vi "MB_Master.vi"() -> ()   [LabVIEW 2015]
doc: "Modbus主机模式"
uses:
  lib/pcomm/PCOMM.lvlib
panel:
  in  "轮询？":bool
  in  "轮询间隔时间":u32=1000 caption="ms" min=30 max=65535 format="%5.0f"
  in  "超时时间":u32=200 caption="ms" min=30 max=65535 format="%5.0f"
  in  "字节数":u16 caption="寄存器值" format="%04x"
  out "LRC8":u8 format="%02x"
  out "CRC16 Hi":u8 format="%02x"
  out "CRC16 Lo":u8 format="%02x"
  in  "数据量":u16 min=1 max=125 format="%04x"
  in  "起始地址":u16 format="%04x"
  in  "功能码":u8(ring)=1 items=["01"=1, "02"=2, "03"=3, "04"=4, "05"=5, "06"=6, "0F"=15, "10"=16]
  in  "从设备编号":u8 format="%02x"
  in  "数据域":u8[](array[numeric]) format="%02x"
  in  "手动发送":bool
  out "接收":string caption="Rx:"
  in  "发送":string caption="Tx:"
  in  "刷新按钮":bool
  in  "字符串":string="串口设置"
  in  "串口号":i32(ring)=1 items=["COM1 通信端口 (COM1)"=1, "COM2 ELTIMA Virtual Serial Port (COM2->COM3)"=2, "COM3 ELTIMA Virtual Serial Port (COM3->COM2)"=3, "COM8 USB-SERIAL CH340 (COM8)"=8]
  in  "奇偶校验":i32(ring)=8 caption="校   验" items=["None"=0, "Odd"=8, "Even"=24, "Mark"=40, "Space"=56]
  in  "数据比特":i32(ring)=3 caption="数据位" items=["5", "6", "7", "8"]
  in  "波特率":i32(ring)=16 items=["1800"=8, "2400"=9, "4800"=10, "7200"=11, "9600"=12, "19200"=13, "38400"=14, "57600"=15, "115200"=16, "230400"=17, "460800"=18, "921600"=19]
  in  "停止位":i32(ring) items=["1"=0, "2"=4]
  in  "打开/关闭串口":bool
  in  "Rx":u32
  in  "Tx":u32
  in  "通信模式":enum16{"RTU", "ASCII"}(ring)
  in  "主从选择":enum32{"Master"}(ring)
  in  "接收帧分析":string
  # "RTU模式不会去检测字符间超时事件"
  # "轮询间隔"
  # "超时时间"
  # "主从模式"
  # "通信模式"
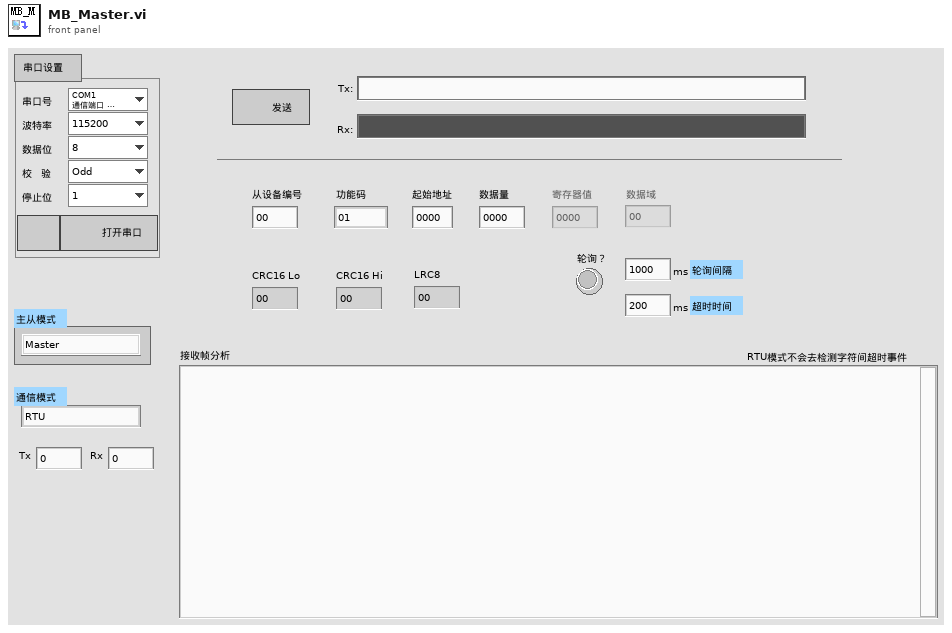
[diagram p1: front panel]
types:
  T1 = enum8{"Enabled", "Disabled", "Disabled and Grayed Out"}
  T2 = typedef "LVRectTypeDef.ctl" = cluster{"Left":i16, "Top":i16, "Right":i16, "Bottom":i16}
  T3 = typedef "LVPointTypeDef.ctl" = cluster{"Horizontal":i16, "Vertical":i16}
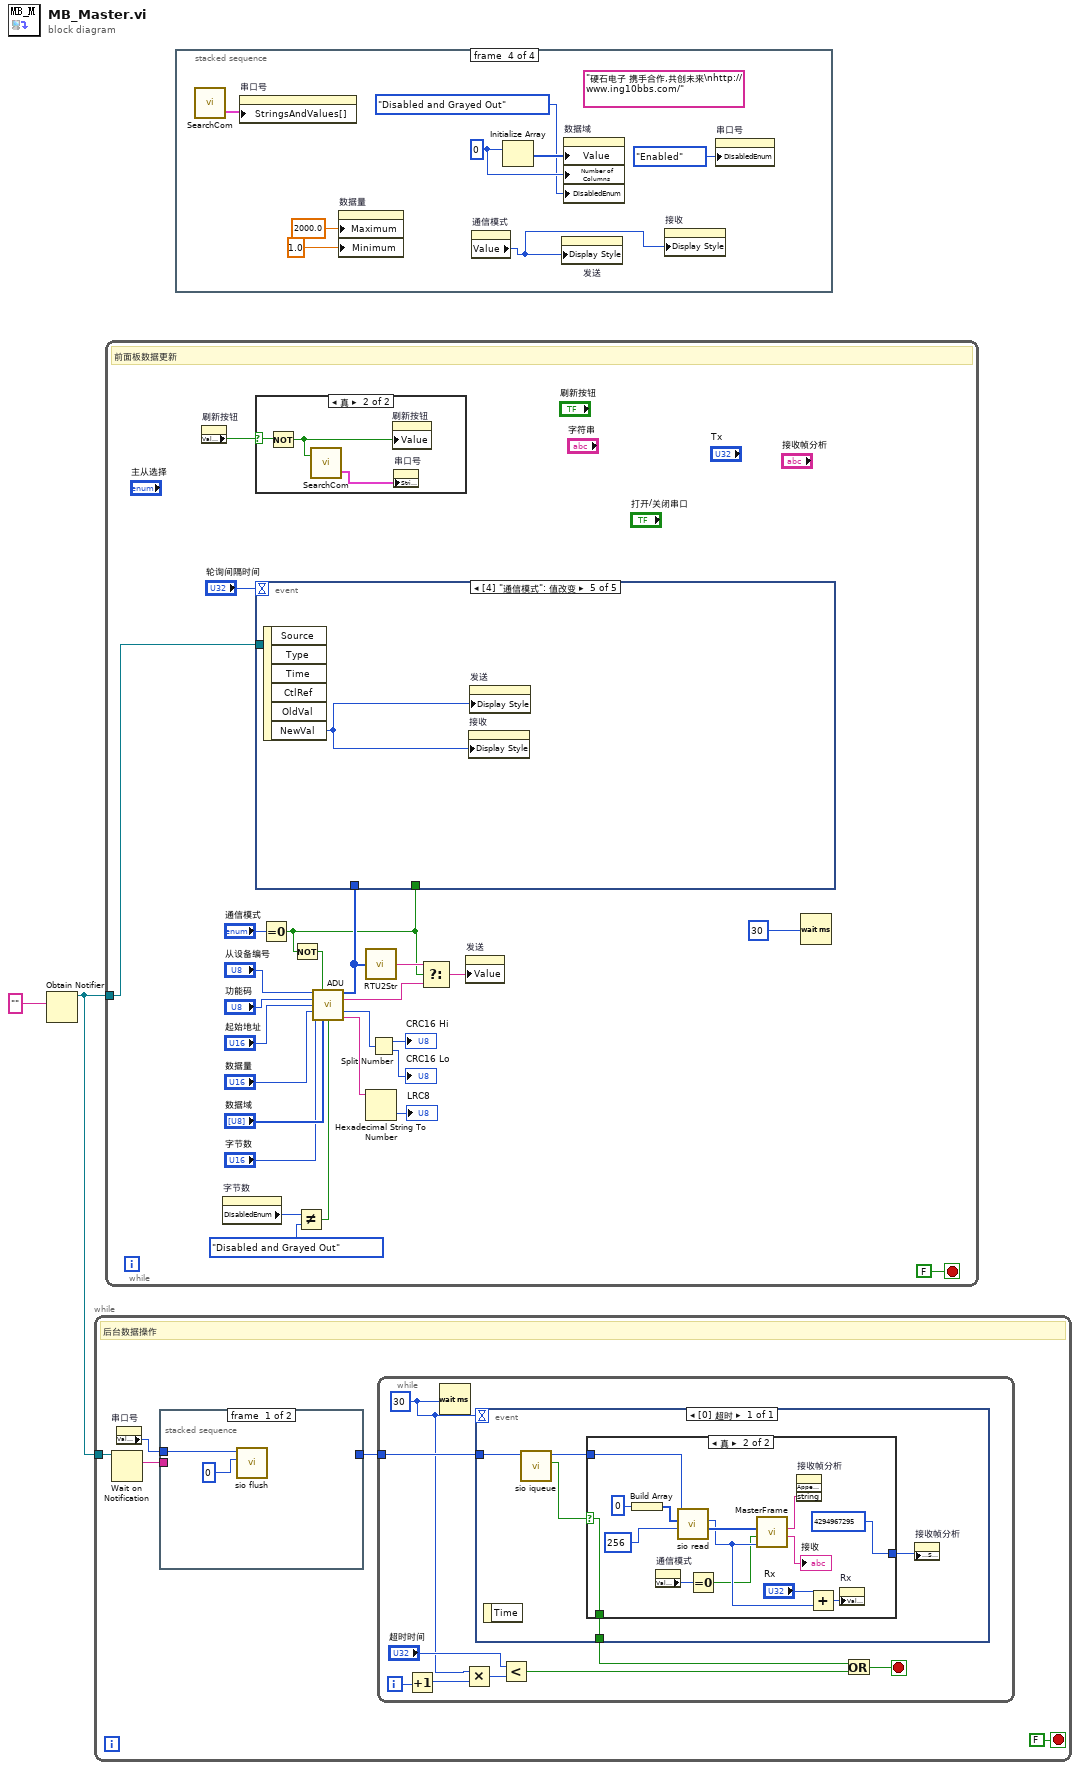
[diagram p0: block diagram]
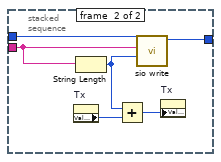
[diagram p2: hidden frame]
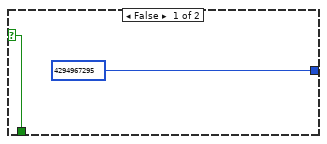
[diagram p3: hidden frame]
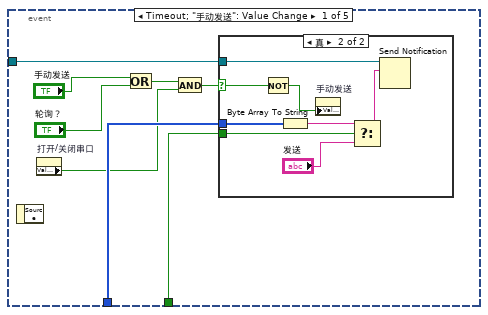
[diagram p4: hidden frame]
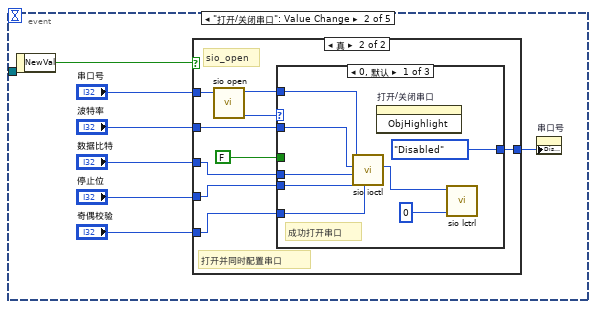
[diagram p6: hidden frame]
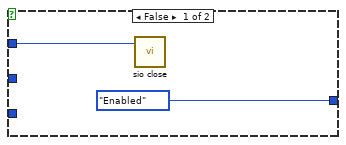
[diagram p7: hidden frame]
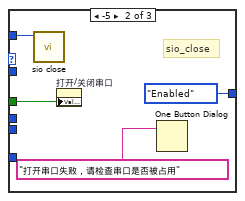
[diagram p8: hidden frame]
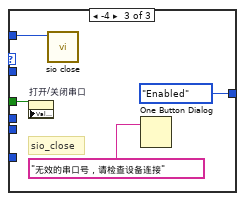
[diagram p9: hidden frame]
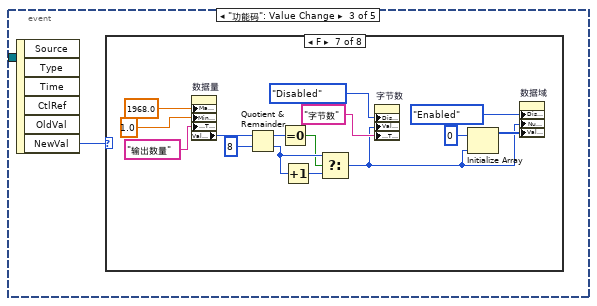
[diagram p10: hidden frame]
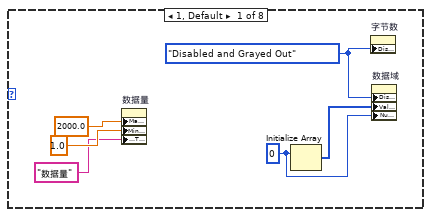
[diagram p11: hidden frame]
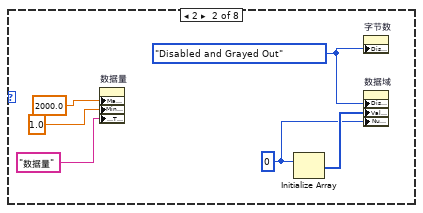
[diagram p12: hidden frame]
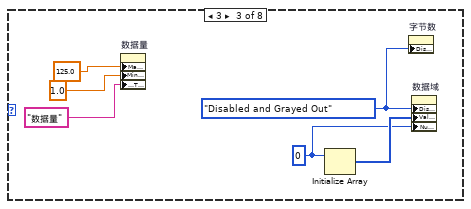
[diagram p13: hidden frame]
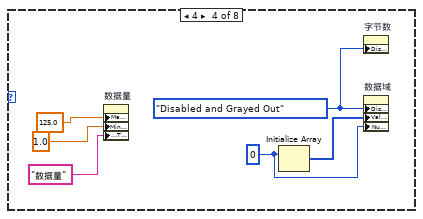
[diagram p14: hidden frame]
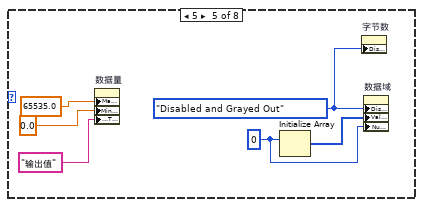
[diagram p15: hidden frame]
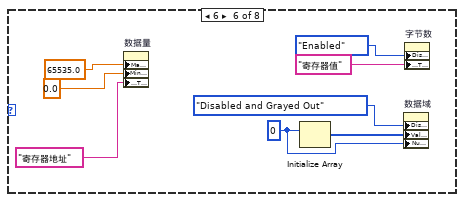
[diagram p16: hidden frame]
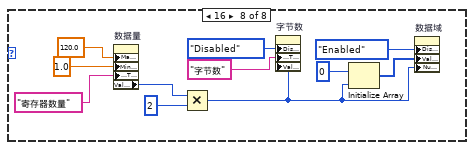
[diagram p17: hidden frame]
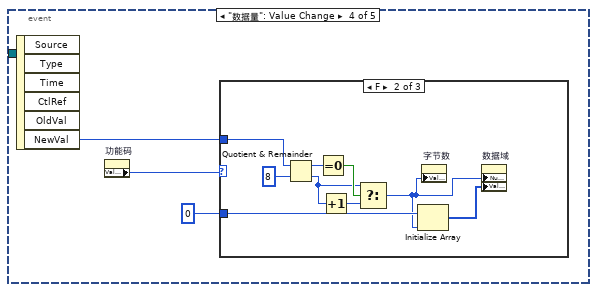
[diagram p18: hidden frame]
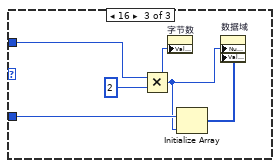
[diagram p20: hidden frame]
diagram:
  n1 = Obtain Notifier(notification data type="") -> (notifier out=w2:refnum<notifier>)  [unwired: 3 in, 2 out]
  n2 = while {
    tunnel: w2 -> [w7]
    stop <- FALSE stop-if-true
    # "后台数据操作"
    n3 = Wait on Notification(notifier=w7) -> (notification=w5:string)  [unwired: 3 in, 3 out]
    n4 = property on="串口号" class="Ring (严格)"() -> ("Value"=w3:i32)  [unwired: 2 in, 2 out]
    n5 = stacked-sequence {
      tunnel: w5 -> [_ w14]
      tunnel: [_ w15] -> w4
      tunnel: w3 -> [w8 w13]
      frame #0 {
        n6 = call "sio flush.vi"("func"=0, "port"=w8) -> ()  [unwired: 8 in, 2 out]
      }
      frame #1 {
        n7 = property on="Tx" class="DigNum (严格)"() -> ("Value"=w11:u32)  [unwired: 2 in, 2 out]
        n8 = String Length(string=w14) -> (length=w12:i32)
        n9 = Add(x=w12, y=w11) -> (x+y=w10:u32)
        n10 = call "sio write.vi"("len"=w12, "buf"=w14, "port"=w13) -> ("port out"=w15:i32)  [unwired: 6 in, 2 out]
        n11 = property on="Tx" class="DigNum (严格)"("Value"=w10) -> ()  [unwired: 2 in, 2 out]
      }
    }
    n12 = while {
      tunnel: w4 -> [w23]
      i -> [w22]
      stop <- w24 stop-if-true
      w16 = 30
      n13 = Increment(x=w22) -> (x+1=w21:i32)
      n14 = Wait (ms)(milliseconds to wait=w16) -> ()  [unwired: 1 out]
      n15 = Multiply(x=w16, y=w21) -> (x*y=w19:i32)
      n16 = event shown="[0] 超时" {
        selector: _ -> [_]
        dyn-events: _ -> [_]
        timeout: w16 -> [_]
        tunnel: w23 -> [w29]
        tunnel: [w27] -> w17
        event Timeout {
          n17 = event-data() -> ()  [unwired: 1 in, 1 out]
          n18 = call "sio iqueue.vi"("port"=w29) -> ("not empty"=w28:bool, "port"=w26:i32)  [unwired: 8 in, 1 out]
          n19 = case shown="真" w28 {
            selector: w28 -> [w31 w41]
            tunnel: w26 -> [_ w42]
            tunnel: [w31 w41] -> w27
            tunnel: [u32 4294967295 u32 4294967295] -> w25
            frame False {
            }
            frame True {
              n20 = Build Array(i8 0) -> (w45:i8[])
              n21 = property on="通信模式" class="Enum (严格)"() -> ("Value"=w36:enum16{"RTU", "ASCII"})  [unwired: 2 in, 2 out]
              n22 = call "sio read.vi"("len"=256, "buf"=w45, "port"=w42) -> ("buf out"=w39:i8[], "Status"=w38:i32)  [unwired: 4 in, 2 out]
              n23 = Equal To 0?(x=w36) -> (x = 0?=w37:bool)
              n24 = call "MasterFrame.vi"("数组大小"=w38, "Mode"=w37, "buf"=w39) -> ("接收显示"=→"接收":string, "数据帧分析"=w40:string)  [unwired: 7 in]
              n25 = invoke on="接收帧分析" class="Str" method="Append String"("string"=w40) -> ()  [unwired: 3 in, 4 out]
              n26 = Add(x="Rx", y=w38) -> (x+y=w33:u32)
              n27 = property on="Rx" class="DigNum (严格)"("Value"=w33) -> ()  [unwired: 2 in, 2 out]
            }
          }
          n28 = property on="接收帧分析" class="Str"("Text.Scroll Position"=w25) -> ()  [unwired: 2 in, 2 out]
        }
      }
      n29 = Less?(x="超时时间", y=w19) -> (x < y?=w18:bool)
      n30 = Or(x=w17, y=w18) -> (x .or. y?=w24:bool)
    }
  }
  n31 = while {
    tunnel: w2 -> [w69]
    stop <- FALSE stop-if-true
    # "前面板数据更新"
    n32 = property on="刷新按钮" class="Bool (严格)"() -> ("Value"=w70:bool)  [unwired: 2 in, 2 out]
    n33 = property on="字节数" class="DigNum (严格)"() -> ("DisabledEnum"=w52:T1)  [unwired: 2 in, 2 out]
    n34 = case shown="真" w70 {
      selector: w70 -> [_ w206]
      frame False {
      }
      frame True {
        n35 = Not(x=w206) -> (.not. x?=w205:bool)
        n36 = call "SearchCom.vi"("使用注册表？"=w205) -> ("下拉列表项"=w207:cluster{"String":string, "Value":i32}[])  [unwired: 2 in]
        n37 = property on="刷新按钮" class="Bool (严格)"("Value"=w205) -> ()  [unwired: 2 in, 2 out]
        n38 = property on="串口号" class="Ring (严格)"("StringsAndValues[]"=w207) -> ()  [unwired: 2 in, 2 out]
      }
    }
    n39 = Equal To 0?(x="通信模式") -> (x = 0?=w46:bool)
    n40 = Not(x=w46) -> (.not. x?=w57:bool)
    n41 = Not Equal?(x=w52, y=T1."Disabled and Grayed Out" ("禁用")) -> (x != y?=w51:bool)
    n42 = call "ADU.vi"("从设备编号"="从设备编号", "ASCII？"=w57, "功能码"="功能码", "起始地址"="起始地址", "数据量"="数据量", "字节数"="字节数", "数据域"="数据域", "字节数？"=w51) -> ("RTU数据帧"=w47:u8[], "ASCII数据帧"=w55:string, "CRC-16"=w67:u16, "LRC-8"=w63:string)  [unwired: 4 in]
    n43 = event shown="[4] \"通信模式\": 值改变" {
      selector: _ -> [_ _ _ _ _]
      dyn-events: _ -> [_ _ _ _ _]
      timeout: "轮询间隔时间" -> [_ _ _ _ _]
      tunnel: w69 -> [w79 _ _ _ _]
      tunnel: w47 -> [w78 _ _ _ _]
      tunnel: w46 -> [w77 _ _ _ _]
      event Timeout; "手动发送": Value Change {
        n44 = event-data() -> ()  [unwired: 1 in, 1 out]
        n45 = property on="打开/关闭串口" class="Bool (严格)"() -> ("Value"=w74:bool)  [unwired: 2 in, 2 out]
        n46 = Or(x="手动发送", y="轮询？") -> (x .or. y?=w73:bool)
        n47 = And(x=w73, y=w74) -> (x .and. y?=w72:bool)
        n48 = case shown="真" w72 {
          selector: w72 -> [_ w85]
          tunnel: w77 -> [_ w87]
          tunnel: w79 -> [_ w86]
          tunnel: w78 -> [_ w80]
          frame False {
          }
          frame True {
            n49 = Not(x=w85) -> (.not. x?=w84:bool)
            n50 = Byte Array To String(unsigned byte array=w80) -> (string=w83:string)
            n51 = property on="手动发送" class="Bool (严格)"("Value"=w84) -> ()  [unwired: 2 in, 2 out]
            n52 = Select(t=w83, s=w87, f="发送") -> (s? t:f=w81:string)
            n53 = Send Notification(notification=w81, notifier=w86) -> ()  [unwired: 1 in, 2 out]
          }
        }
      }
      event "打开/关闭串口": Value Change {
        n54 = event-data() -> ("NewVal"=w93:bool)  [unwired: 1 in]
        n55 = case shown="真" w93 {
          tunnel: [T1."Enabled" w105] -> w94
          tunnel: "串口号" -> [w95 w104]
          tunnel: "奇偶校验" -> [_ w100]
          tunnel: "停止位" -> [_ w99]
          tunnel: "数据比特" -> [_ w98]
          tunnel: "波特率" -> [_ w97]
          frame False {
            n56 = call "sio close.vi"("port"=w95) -> ()  [unwired: 9 in, 2 out]
          }
          frame True {
            # "sio_open"
            # "打开并同时配置串口"
            n57 = call "sio open.vi"("port"=w104) -> ("port"=w103:i32, "Status"=w102:i32)  [unwired: 6 in]
            n58 = case shown="0, 默认" w102 {
              tunnel: w103 -> [w112 w115 w119]
              tunnel: [T1."Disabled" T1."Enabled" T1."Enabled"] -> w105
              tunnel: FALSE -> [_ w114 w118]
              tunnel: w100 -> [w111 _ _]
              tunnel: w99 -> [w110 _ _]
              tunnel: w98 -> [w109 _ _]
              tunnel: w97 -> [w108 _ _]
              frame 0, Default {
                # "成功打开串口"
                n59 = call "sio ioctl.vi"("parity"=w111, "stop bits"=w110, "data bits"=w109, "baud"=w108, "port"=w112) -> ("port"=w107:i32)  [unwired: 5 in, 1 out]
                n60 = invoke on="打开/关闭串口" class="Bool (严格)" method="ObjHighlight"() -> ()  [unwired: 3 in, 3 out]
                n61 = call "sio lctrl.vi"("mode"=0, "port"=w107) -> ()  [unwired: 8 in, 2 out]
              }
              frame -5 {
                # "sio_close"
                n62 = call "sio close.vi"("port"=w115) -> ()  [unwired: 9 in, 2 out]
                n63 = property on="打开/关闭串口" class="Bool (严格)"("Value"=w114) -> ()  [unwired: 2 in, 2 out]
                n64 = One Button Dialog(message="打开串口失败，请检查串口是否被占用") -> ()  [unwired: 1 in, 1 out]
              }
              frame -4 {
                # "sio_close"
                n65 = property on="打开/关闭串口" class="Bool (严格)"("Value"=w118) -> ()  [unwired: 2 in, 2 out]
                n66 = call "sio close.vi"("port"=w119) -> ()  [unwired: 9 in, 2 out]
                n67 = One Button Dialog(message="无效的串口号，请检查设备连接") -> ()  [unwired: 1 in, 1 out]
              }
            }
          }
        }
        n68 = property on="串口号" class="Ring (严格)"("DisabledEnum"=w94) -> ()  [unwired: 2 in, 2 out]
      }
      event "功能码": Value Change {
        n69 = event-data() -> ("NewVal"=w122:u8)  [unwired: 1 in, 5 out]
        n70 = case shown="F" w122 {
          frame 1, Default {
            w123 = u8 0 ("值")
            w126 = T1."Disabled and Grayed Out" ("禁用")
            n71 = property on="数据量" class="DigNum (严格)"("Maximum"=2000.0, "Minimum"=1.0, "Caption.Text"="数据量") -> ()  [unwired: 2 in, 2 out]
            n72 = Initialize Array(w123) -> (w124:u8[])  [unwired: 1 in]
            n73 = property on="字节数" class="DigNum (严格)"("DisabledEnum"=w126) -> ()  [unwired: 2 in, 2 out]
            n74 = property on="数据域" class="Arr (严格)"("DisabledEnum"=w126, "Value"=w124, "Number of Columns"=w123) -> ()  [unwired: 2 in, 2 out]
          }
          frame 2 {
            w129 = u8 0 ("值")
            w132 = T1."Disabled and Grayed Out" ("禁用")
            n75 = property on="数据量" class="DigNum (严格)"("Maximum"=2000.0, "Minimum"=1.0, "Caption.Text"="数据量") -> ()  [unwired: 2 in, 2 out]
            n76 = Initialize Array(w129) -> (w130:u8[])  [unwired: 1 in]
            n77 = property on="字节数" class="DigNum (严格)"("DisabledEnum"=w132) -> ()  [unwired: 2 in, 2 out]
            n78 = property on="数据域" class="Arr (严格)"("DisabledEnum"=w132, "Value"=w130, "Number of Columns"=w129) -> ()  [unwired: 2 in, 2 out]
          }
          frame 3 {
            w135 = u8 0 ("值")
            w138 = T1."Disabled and Grayed Out" ("禁用")
            n79 = property on="数据量" class="DigNum (严格)"("Maximum"=125.0, "Minimum"=1.0, "Caption.Text"="数据量") -> ()  [unwired: 2 in, 2 out]
            n80 = Initialize Array(w135) -> (w136:u8[])  [unwired: 1 in]
            n81 = property on="字节数" class="DigNum (严格)"("DisabledEnum"=w138) -> ()  [unwired: 2 in, 2 out]
            n82 = property on="数据域" class="Arr (严格)"("DisabledEnum"=w138, "Value"=w136, "Number of Columns"=w135) -> ()  [unwired: 2 in, 2 out]
          }
          frame 4 {
            w141 = u8 0 ("值")
            w144 = T1."Disabled and Grayed Out" ("禁用")
            n83 = property on="数据量" class="DigNum (严格)"("Maximum"=125.0, "Minimum"=1.0, "Caption.Text"="数据量") -> ()  [unwired: 2 in, 2 out]
            n84 = Initialize Array(w141) -> (w142:u8[])  [unwired: 1 in]
            n85 = property on="字节数" class="DigNum (严格)"("DisabledEnum"=w144) -> ()  [unwired: 2 in, 2 out]
            n86 = property on="数据域" class="Arr (严格)"("DisabledEnum"=w144, "Value"=w142, "Number of Columns"=w141) -> ()  [unwired: 2 in, 2 out]
          }
          frame 5 {
            w147 = u8 0 ("值")
            w150 = T1."Disabled and Grayed Out" ("禁用")
            n87 = property on="数据量" class="DigNum (严格)"("Maximum"=65535.0 ("数据输入界限:最大值"), "Minimum"=0.0, "Caption.Text"="输出值") -> ()  [unwired: 2 in, 2 out]
            n88 = Initialize Array(w147) -> (w148:u8[])  [unwired: 1 in]
            n89 = property on="字节数" class="DigNum (严格)"("DisabledEnum"=w150) -> ()  [unwired: 2 in, 2 out]
            n90 = property on="数据域" class="Arr (严格)"("DisabledEnum"=w150, "Value"=w148, "Number of Columns"=w147) -> ()  [unwired: 2 in, 2 out]
          }
          frame 6 {
            w155 = u8 0 ("值")
            n91 = property on="数据量" class="DigNum (严格)"("Maximum"=65535.0 ("数据输入界限:最大值"), "Minimum"=0.0, "Caption.Text"="寄存器地址") -> ()  [unwired: 2 in, 2 out]
            n92 = Initialize Array(w155) -> (w156:u8[])  [unwired: 1 in]
            n93 = property on="数据域" class="Arr (严格)"("DisabledEnum"=T1."Disabled and Grayed Out" ("禁用"), "Value"=w156, "Number of Columns"=w155) -> ()  [unwired: 2 in, 2 out]
            n94 = property on="字节数" class="DigNum (严格)"("DisabledEnum"=T1."Enabled" ("禁用"), "Caption.Text"="寄存器值") -> ()  [unwired: 2 in, 2 out]
          }
          frame 15 {
            n95 = property on="数据量" class="DigNum (严格)"("Maximum"=1968.0 ("数据输入界限:最大值"), "Minimum"=1.0, "Caption.Text"="输出数量") -> ("Value"=w162:u16)  [unwired: 2 in, 2 out]
            n96 = Quotient & Remainder(x=w162, y=u16 8) -> (x-y*floor(x/y)=w169:u16, floor(x/y)=w168:u16)
            n97 = Equal To 0?(x=w169) -> (x = 0?=w167:bool)
            n98 = Increment(x=w168) -> (x+1=w166:u16)
            n99 = Select(t=w168, s=w167, f=w166) -> (s? t:f=w161:u16)
            n100 = property on="字节数" class="DigNum (严格)"("DisabledEnum"=T1."Disabled" ("禁用"), "Value"=w161, "Caption.Text"="字节数") -> ()  [unwired: 2 in, 2 out]
            n101 = Initialize Array(u8 0 ("值"), w161) -> (w165:u8[])
            n102 = property on="数据域" class="Arr (严格)"("DisabledEnum"=T1."Enabled" ("禁用"), "Number of Columns"=w161, "Value"=w165) -> ()  [unwired: 2 in, 2 out]
          }
          frame 16 {
            n103 = property on="数据量" class="DigNum (严格)"("Maximum"=120.0 ("数据输入界限:最大值"), "Minimum"=1.0, "Caption.Text"="寄存器数量") -> ("Value"=w178:u16)  [unwired: 2 in, 2 out]
            n104 = Multiply(x=w178, y=u16 2) -> (x*y=w176:u16)
            n105 = property on="字节数" class="DigNum (严格)"("DisabledEnum"=T1."Disabled" ("禁用"), "Caption.Text"="字节数", "Value"=w176) -> ()  [unwired: 2 in, 2 out]
            n106 = Initialize Array(u8 0 ("值"), w176) -> (w182:u8[])
            n107 = property on="数据域" class="Arr (严格)"("DisabledEnum"=T1."Enabled" ("禁用"), "Value"=w182, "Number of Columns"=w176) -> ()  [unwired: 2 in, 2 out]
          }
        }
      }
      event "数据量": Value Change {
        n108 = event-data() -> ("NewVal"=w188:u16)  [unwired: 1 in, 5 out]
        n109 = property on="功能码" class="Ring (严格)"() -> ("Value"=w189:u8)  [unwired: 2 in, 2 out]
        n110 = case shown="F" w189 {
          tunnel: w188 -> [_ w193 w202]
          tunnel: u8 0 -> [_ w192 w201]
          frame 0, Default {
          }
          frame 15 {
            n111 = Quotient & Remainder(x=w193, y=u16 8) -> (x-y*floor(x/y)=w195:u16, floor(x/y)=w196:u16)
            n112 = Equal To 0?(x=w195) -> (x = 0?=w197:bool)
            n113 = Increment(x=w196) -> (x+1=w198:u16)
            n114 = Select(t=w196, s=w197, f=w198) -> (s? t:f=w190:u16)
            n115 = Initialize Array(w192, w190) -> (w191:u8[])
            n116 = property on="字节数" class="DigNum (严格)"("Value"=w190) -> ()  [unwired: 2 in, 2 out]
            n117 = property on="数据域" class="Arr (严格)"("Number of Columns"=w190, "Value"=w191) -> ()  [unwired: 2 in, 2 out]
          }
          frame 16 {
            n118 = Multiply(x=w202, y=u16 2) -> (x*y=w200:u16)
            n119 = property on="字节数" class="DigNum (严格)"("Value"=w200) -> ()  [unwired: 2 in, 2 out]
            n120 = Initialize Array(w201, w200) -> (w199:u8[])
            n121 = property on="数据域" class="Arr (严格)"("Number of Columns"=w200, "Value"=w199) -> ()  [unwired: 2 in, 2 out]
          }
        }
      }
      event "通信模式": Value Change {
        n122 = event-data() -> ("NewVal"=w204:enum16{"RTU", "ASCII"})  [unwired: 1 in, 5 out]
        n123 = property on="接收" class="Str"("Display Style"=w204) -> ()  [unwired: 2 in, 2 out]
        n124 = property on="发送" class="Str"("Display Style"=w204) -> ()  [unwired: 2 in, 2 out]
      }
    }
    n125 = call "RTU2Str.vi"("RTU数据帧"=w47) -> ("RTU数据帧字符串"=w56:string)
    n126 = Hexadecimal String To Number(string=w63) -> (number=→"LRC8":u32)  [unwired: 2 in, 1 out]
    n127 = Split Number(x=w67) -> (hi(x)=→"CRC16 Hi":u8, lo(x)=→"CRC16 Lo":u8)
    n128 = Select(t=w56, s=w46, f=w55) -> (s? t:f=w59:string)
    n129 = property on="发送" class="Str"("Value"=w59) -> ()  [unwired: 2 in, 2 out]
    n130 = Wait (ms)(milliseconds to wait=30) -> ()  [unwired: 1 out]
  }
  n131 = stacked-sequence {
    frame #0 {
      n132 = Wait (ms)(milliseconds to wait=u32 20) -> ()  [unwired: 1 out]
    }
    frame #1 {
      # "调整启动时的前面板尺寸边界"
      # "应当等程序启动之后再执行这一步→_→"
      n133 = Call Chain ("调用链")() -> (call chain=w214:string[])
      n134 = Index Array(array=w214, index=0) -> (element=w212:string)
      n135 = Open VI Reference(vi path=w212) -> (vi reference=w223:refnum<vi>)  [unwired: 1 in, 5 out]
      n136 = property class="VI"(reference=w223) -> ("Front Panel.PanelBounds"=w220:T2)  [unwired: 1 in, 2 out]
      n137 = property class="VI"(reference=w223) -> (reference out=w209:refnum<vi>, "Minimum Panel Size"=w215:T3)  [unwired: 1 in, 1 out]
      n138 = Unbundle By Name(w215) -> ("Horizontal"=w221:i16, "Vertical"=w218:i16)
      n139 = Unbundle By Name(w220) -> ("Left"=w222:i16, "Top"=w217:i16)
      n140 = Add(x=w221, y=w222) -> (x+y=w219:i16)
      n141 = Add(x=w218, y=w217) -> (x+y=w216:i16)
      n142 = Bundle By Name(cluster=w220, "Right"=w219, "Bottom"=w216) -> (w211:T2)
      n143 = property class="VI"(reference=w209, "Front Panel.PanelBounds"=w211) -> (reference out=w210:refnum<vi>)  [unwired: 1 in, 1 out]
      n144 = Close Reference(reference=w210) -> ()  [unwired: 1 in, 1 out]
    }
    frame #2 {
      w226 = i16 0
      # "自动调整窗格原点"
      n145 = property on="窗格" class="Pane"() -> ("Origin"=w225:T3)  [unwired: 2 in, 2 out]
      n146 = Bundle By Name(cluster=w225, "Horizontal"=w226, "Vertical"=w226) -> (w224:T3)
      n147 = property on="窗格" class="Pane"("Origin"=w224) -> ()  [unwired: 2 in, 2 out]
    }
    frame #3 {
      w230 = u8 0 ("值")
      (unwired) "硬石电子 携手合作,共创未来\nhttp://www.ing10bbs.com/"
      n148 = call "SearchCom.vi"() -> ("下拉列表项"=w234:cluster{"String":string, "Value":i32}[])  [unwired: 3 in]
      n149 = property on="串口号" class="Ring (严格)"("StringsAndValues[]"=w234) -> ()  [unwired: 2 in, 2 out]
      n150 = property on="数据量" class="DigNum (严格)"("Maximum"=2000.0, "Minimum"=1.0) -> ()  [unwired: 2 in, 2 out]
      n151 = property on="通信模式" class="Enum (严格)"() -> ("Value"=w227:enum16{"RTU", "ASCII"})  [unwired: 2 in, 2 out]
      n152 = Initialize Array(w230) -> (w231:u8[])  [unwired: 1 in]
      n153 = property on="发送" class="Str"("Display Style"=w227) -> ()  [unwired: 2 in, 2 out]
      n154 = property on="数据域" class="Arr (严格)"("Value"=w231, "Number of Columns"=w230, "DisabledEnum"=T1."Disabled and Grayed Out" ("禁用")) -> ()  [unwired: 2 in, 2 out]
      n155 = property on="接收" class="Str"("Display Style"=w227) -> ()  [unwired: 2 in, 2 out]
      n156 = property on="串口号" class="Ring (严格)"("DisabledEnum"=T1."Enabled" ("禁用")) -> ()  [unwired: 2 in, 2 out]
    }
  }
